vi "Read Video High Resolution Dani.vi"(8 "error in (no error)":errorcluster, 10 "video":u32[](array[numeric]), 11 "Image In":T1) -> (0 "error out":errorcluster, 3 "Image Out":T1)   [LabVIEW 2015]
uses:
  <vilib>/vision/Image Controls.llb/IMAQ Image.ctl
  libkinect_wrapper.dll
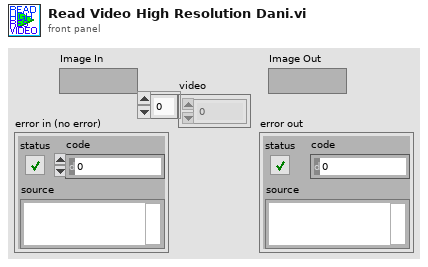
[diagram p1: front panel]
types:
  T1 = typedef "IMAQ Image.ctl" = refnum<image>
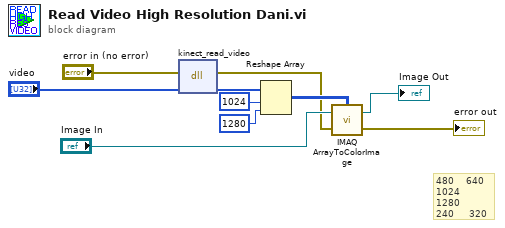
[diagram p0: block diagram]
diagram:
  # "480    640\n1024   1280\n240     320"
  n1 = dll-call lib="libkinect_wrapper.*" fn="kinect_read_video"(error in="error in (no error)", "video"="video") -> (error out=w3:errorcluster, "video"=w8:u32[])  [unwired: 3 in, 1 out]
  n2 = Reshape Array(w8, 1024 ("dimension size"), 1280 ("dimension size")) -> (w5:u32[][])
  n3 = call "IMAQ ArrayToColorImage"("Image Pixels (U32)"=w5, "Image"="Image In", "error in (no error)"=w3) -> ("Image Out"=→"Image Out":T1, "error out"=→"error out":errorcluster)  [unwired: 2 in]
